vi "Clock.vi"() -> ()   [LabVIEW 2019]
uses:
  <vilib>/eio/EIONode/EIONode.xnode
  <vilib>/rvi/eio/common/nirviEmuTemplateMethod_errors.vi
panel:
  in  "stop":bool
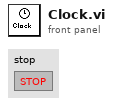
[diagram p1: front panel]
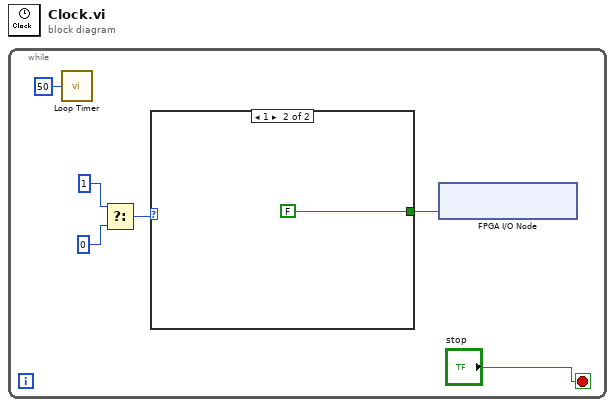
[diagram p0: block diagram]
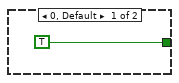
[diagram p2: hidden frame]
diagram:
  n1 = while {
    stop <- "stop" stop-if-true
    n2 = call "Loop Timer"("Count(mSec)"=u32 50) -> ()  [unwired: 1 out]
    n3 = Select(t=i16 1, f=i16 0) -> (s? t:f=w5:i16)  [unwired: 1 in]
    n4 = case shown="1" w5 {
      tunnel: [TRUE FALSE] -> w4
      frame 0, Default {
      }
      frame 1 {
      }
    }
    n5 = xnode "FPGA I/O Node"("ConnectorA/DIO0"=w4) -> ()  [unwired: 1 in, 1 out]
  }
